vi "Detect Send Rising Edge.vi"(11 "OOB to Logic Data in":T1 {"Payload LIN" format="%x"; "ID LIN" format="%x"; "Payload CAN" format="%x"; "Type CAN" items=["CAN Data"=0, "CAN Remote"=1, "CAN Bus Error"=2, "CAN 2.0 Data"=8, "CAN FD Data"=16, "CAN FD+BRS Data"=24, "J1939 Data"=192, "Delay"=224, "Log Trigger"=225, "Start Trigger"=226]; "ID CAN" format="%x"}) -> (3 "crossing":bool)   [LabVIEW 2025, in "CAN-LIN Frame Generator.lvclass"]
uses:
  CAN-LIN Frame Generator.lvclass
  CAN-LIN Frame Generator.lvclass/CAN-LIN Frame Generator.ctl
  <vilib>/ptbypt/NI_PtbyPt.lvlib
  <vilib>/xnet/xnet.llb/XNET Frame Type CAN.ctl
  OOB Data Transfer/Typdefs/OOB to Logic Data.ctl
  OOB Data Transfer/OOB Data Transfer.lvlib
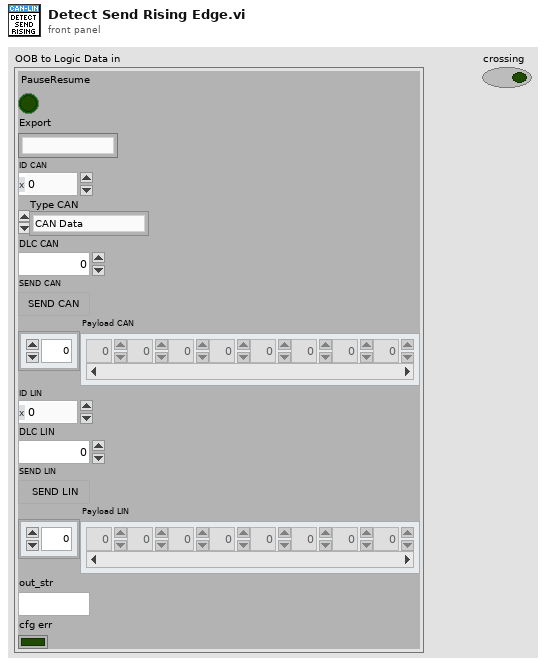
[diagram p1: front panel]
types:
  T1 = typedef "OOB Data Transfer.lvlib/OOB to Logic Data.ctl" = cluster{"PauseResume":bool, "Export":string, "ID CAN":u32, "Type CAN":T2, "DLC CAN":u32, "SEND CAN":bool, "Payload CAN":u32[], "ID LIN":u32, "DLC LIN":u32, "SEND LIN":bool, "Payload LIN":u32[], "out_str":string, "cfg err":bool}
  T2 = typedef "XNET Frame Type CAN.ctl" = u8
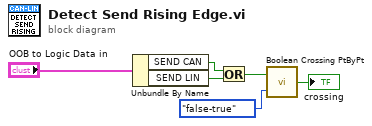
[diagram p0: block diagram]
diagram:
  n1 = Unbundle By Name("OOB to Logic Data in") -> ("SEND CAN"=w2:bool, "SEND LIN"=w3:bool)
  n2 = Or(x=w2, y=w3) -> (x .or. y?=w5:bool)
  n3 = call <vilib>:"Boolean Crossing PtByPt.vi"("direction"=enum16{"either", "false-true", "true-false"}."false-true", "input"=w5) -> ("crossing"=→"crossing":bool)  [unwired: 1 in]
